vi "CustomStartService.vi"(8 "error in":errorcluster, 11 "Server Address":string="localhost:50051") -> (0 "error out":errorcluster, 1 "Listening Port":i32, 2 "Server Stop":refnum<user-event>, 3 "gRPC Server out":refnum<class "Servicer.lvclass">, 5 "MicronUE":refnum<user-event>)   [LabVIEW 2019, in "MicronGRPCGeneratedServer.lvlib"]
uses:
  MicronGRPCGeneratedServer.lvlib
  <vilib>/gRPC/LabVIEW gRPC Servicer/Servicer/Servicer.lvclass
  Base/Server/Message/MessageBase.lvclass
  <vilib>/gRPC/LabVIEW gRPC Servicer/Servicer/Servicer.lvclass/Servicer.ctl
  RPC Service/MicronGRPC/MicronGRPC.lvclass
  C:/Program Files (x86)/National Instruments/LabVIEW 2019/vi.lib/gRPC/LabVIEW gRPC Servicer/ServiceBase/ServiceBase.lvclass
  SubVIs/CustomEventHandler.vi
panel:
  in  "Server Certificate File (.crt)":path
  in  "Server Key File (.key)":path
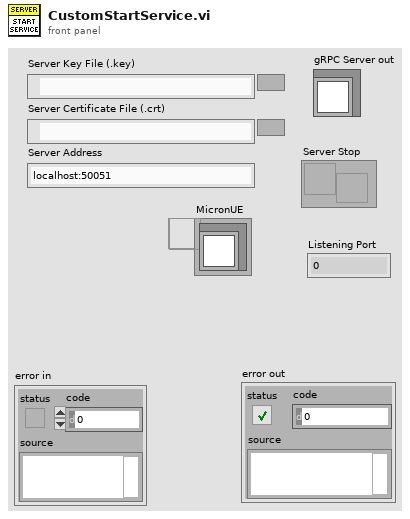
[diagram p1: front panel]
types:
  T1 = typedef "grpc-lvsupport-release.lvlib/grpcId.ctl" = u64
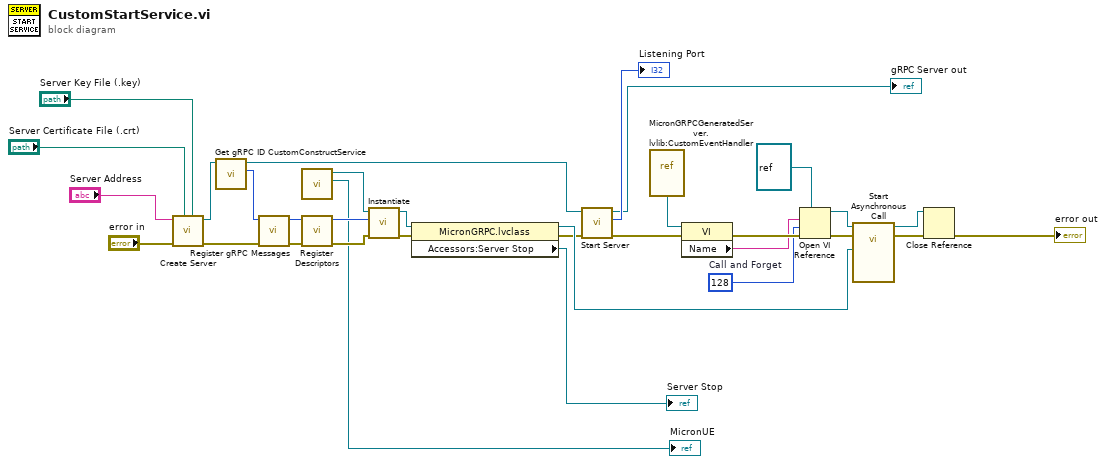
[diagram p0: block diagram]
diagram:
  w5 = 128  # Call and Forget
  n1 = call <vilib>:"Create Server.vi"("Server Key File (.key)"="Server Key File (.key)", "Server Certificate File (.crt)"="Server Certificate File (.crt)", "error in"="error in", "Server Address"="Server Address") -> ("error out"=w26:errorcluster, "gRPC server out"=w28:refnum<class "Servicer.lvclass">)  [unwired: 6 in]
  n2 = call <vilib>:"Get gRPC ID.vi"("gRPC server in"=w28) -> ("gRPC ID"=w27:T1, "gRPC server out"=w23:refnum<class "Servicer.lvclass">)  [unwired: 9 in]
  n3 = call "Register gRPC Messages.vi"("error in (no error)"=w26, "gRPC ID"=w27) -> ("error out"=w25:errorcluster, "gRPC ID Out"=w24:T1)  [unwired: 8 in]
  n4 = call "CustomConstructService.vi"() -> ("MicronMessageUE"=→"MicronUE":refnum<user-event>, "MicronGRPC out"=w18:refnum<class "MicronGRPC.lvclass">)  [unwired: 10 in]
  n5 = call "Register Descriptors.vi"("error in (no error)"=w25, "gRPC ID"=w24) -> ("error out"=w22:errorcluster, "gRPC ID Out"=w21:T1)  [unwired: 8 in]
  n6 = call-dynamic "Instantiate.vi"("error in"=w22, "gRPCid"=w21, "gRPC service in"=w18) -> ("error out"=w19:errorcluster, "gRPC service out"=w20:refnum<class "MicronGRPC.lvclass">)  [unwired: 7 in]
  n7 = property class="MicronGRPC.lvclass"(reference=w20, error in=w19) -> (reference out=w17:refnum<class "MicronGRPC.lvclass">, error out=w16:errorcluster, "Accessors:Server Stop"=→"Server Stop":refnum<user-event>)
  n8 = call <vilib>:"Start Server.vi"("error in"=w16, "gRPC server in"=w23) -> ("error out"=w6:errorcluster, "Listening Port"=→"Listening Port":i32, "gRPC server out"=→"gRPC Server out":refnum<class "Servicer.lvclass">)  [unwired: 7 in]
  n9 = vi-ref "MicronGRPCGeneratedServer.lvlib:CustomEventHandler.vi"() -> (w4:refnum<vi>)
  n10 = property class="VI"(reference=w4, error in=w6) -> (error out=w9:errorcluster, "Name"=w8:string)  [unwired: 1 out]
  n11 = Open VI Reference(type specifier VI Refnum (for type only)=refnum<vi> refnum ("reference"), vi path=w8, options=w5, error in (no error)=w9) -> (vi reference=w10:refnum<vi>, error out=w11:errorcluster)  [unwired: 2 in]
  n12 = call-by-ref "Start Asynchronous Call"(reference=w10, error in=w11, "MicronGRPC.lvclass"=w17) -> (reference out=w1:refnum<vi>, error out=w13:errorcluster)  [unwired: 11 in]
  n13 = Close Reference(reference=w1, error in (no error)=w13) -> (error out=→"error out":errorcluster)
